vi "Post-Build Action.vi"(5 "Files Generated by Build":path[](array[path]), 6 "Top Level/Always Included VIs":path[](array[path]), 7 "Destination Path":path, 8 "error in (no error)":errorcluster, 9 "Target Name":string, 10 "Build Specification Name":string, 11 "Project Path":path) -> (0 "error out":errorcluster)   [LabVIEW 2011]
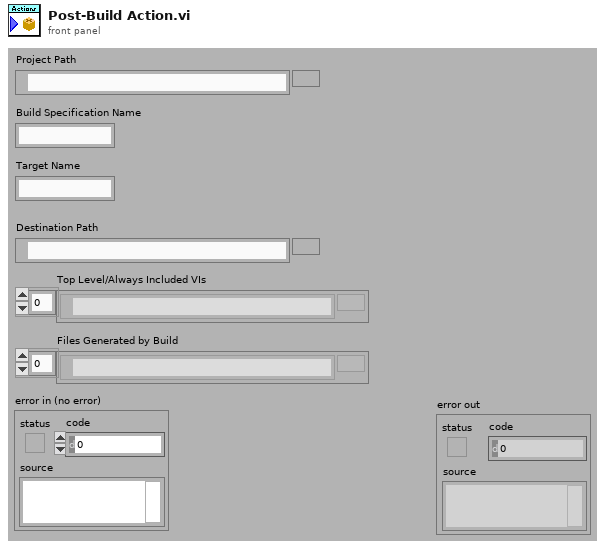
[diagram p1: front panel]
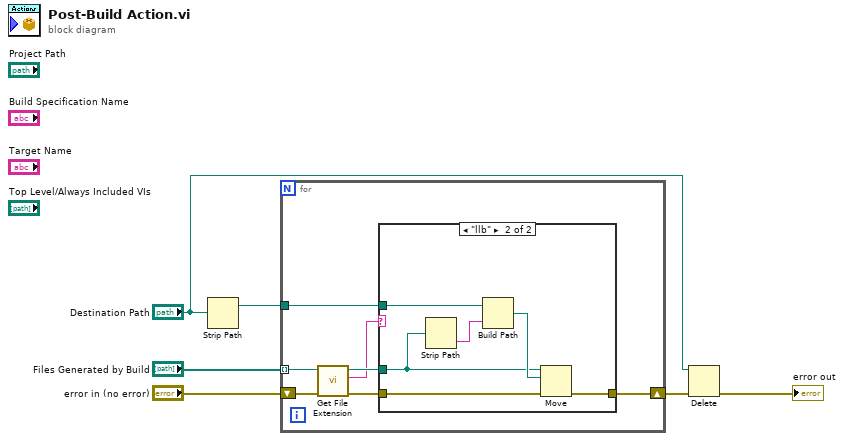
[diagram p0: block diagram]
diagram:
  n1 = Strip Path(path="Destination Path") -> (stripped path=w1:path)  [unwired: 1 out]
  n2 = for {
    tunnel: "Files Generated by Build" -> [w9] mode=indexing
    tunnel: w1 -> [w13]
    shift-right: [w12] -> w4
    shift-left: "error in (no error)" -> [w11]
    n3 = call <vilib>:"Get File Extension.vi"("error in (no error)"=w11, "file"=w9) -> ("error out"=w10:errorcluster, "lowercase file extension"=w7:string, "dup file"=w8:path)  [unwired: 6 in, 1 out]
    n4 = case shown="\"llb\"" w7 {
      tunnel: w13 -> [_ w19]
      tunnel: [w14 w17] -> w12
      tunnel: w10 -> [w14 w16]
      tunnel: w8 -> [_ w15]
      frame Default {
      }
      frame "llb" {
        n5 = Strip Path(path=w15) -> (name=w20:string)  [unwired: 1 out]
        n6 = Build Path(base path=w19, name or relative path=w20) -> (appended path=w18:path)
        n7 = Move(source path=w15, error in=w16, 10:w18) -> (error out=w17:errorcluster)  [unwired: 2 in, 2 out]
      }
    }
  }
  n8 = Delete(path (use dialog)="Destination Path", error in=w4) -> (error out=→"error out":errorcluster)  [unwired: 3 in, 2 out]
